vi "Window Flattop248D.vi"(1 "Normalize? (False)":bool, 2 "N":i32) -> (0 "window":dbl[](array[numeric]))   [LabVIEW 2020, in "FFTWDLL.lvlib"]
doc: "Flattop 248D window (-248dB side lobes)."
uses:
  FFTWDLL.lvlib
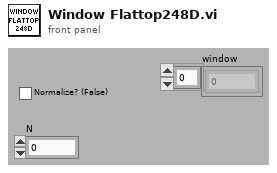
[diagram p1: front panel]
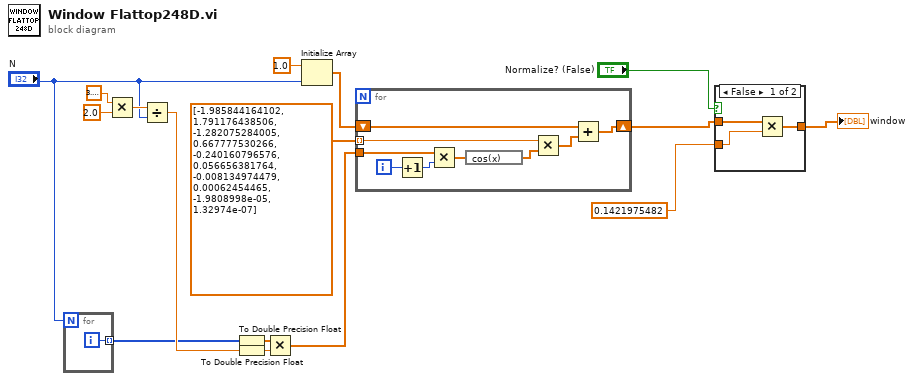
[diagram p0: block diagram]
diagram:
  n1 = for {
    N: "N" -> [_]
    tunnel: [w17] -> w10 mode=indexing
    i -> [w17]
  }
  n2 = Multiply(x=3.141592653589793, y=2.0) -> (x*y=w14:dbl)
  n3 = Divide(x=w14, y="N") -> (x/y=w11:dbl)
  n4 = To Double Precision Float(number=w10) -> (double precision float=w9:dbl[])
  n5 = To Double Precision Float(number=w11) -> (double precision float=w15:dbl)
  n6 = Multiply(x=w9, y=w15) -> (x*y=w16:dbl[])
  n7 = Initialize Array(1.0 ("element"), "N") -> (w8:dbl[])
  n8 = for {
    shift-right: [w23] -> w1
    shift-left: w8 -> [w22]
    tunnel: dbl[] [-1.985844164102, 1.791176438506, -1.282075284005, 0.667777530266, -0.240160796576, 0.056656381764, -0.008134974479, 0.00062454465, -1.9808998e-05, 1.32974e-07] -> [w20] mode=indexing
    tunnel: w16 -> [w18]
    i -> [w24]
    n9 = Increment(x=w24) -> (x+1=w25:i32)
    n10 = Multiply(x=w18, y=w25) -> (x*y=w26:dbl[])
    n11 = expression code="cos(x)"(w26) -> (w21:dbl[])
    n12 = Multiply(x=w20, y=w21) -> (x*y=w19:dbl[])
    n13 = Add(x=w22, y=w19) -> (x+y=w23:dbl[])
  }
  n14 = case shown="False" "Normalize? (False)" {
    tunnel: w1 -> [w29 w30]
    tunnel: [w28 w30] -> w4
    tunnel: 0.1421975482 ("value") -> [w27 _]
    frame False {
      n15 = Multiply(x=w29, y=w27) -> (x*y=w28:dbl[])
    }
    frame True {
    }
  }
  "window" <- w4
